vi "Do.vi"(8 "error in (no error)":errorcluster, 10 "Actor in":refnum<class "Actor.lvclass">, 11 "Linear Actuator Control Task Msg":refnum<class "Linear Actuator Control Task Msg.lvclass">) -> (0 "error out":errorcluster, 2 "Actor out":refnum<class "Actor.lvclass">)   [LabVIEW 2018, in "Linear Actuator Control Actor.lvlib" / "Linear Actuator Control Task Msg.lvclass"]
uses:
  Linear Actuator Control Task Msg.lvclass
  <vilib>/ActorFramework/Actor/Actor.lvclass
  Linear Actuator Control/Linear Actuator Control.lvclass
  C:/Program Files (x86)/National Instruments/LabVIEW 2018/vi.lib/ActorFramework/Actor/Actor.lvclass
  Linear Actuator Control Task Msg.lvclass/Linear Actuator Control Task Msg.ctl
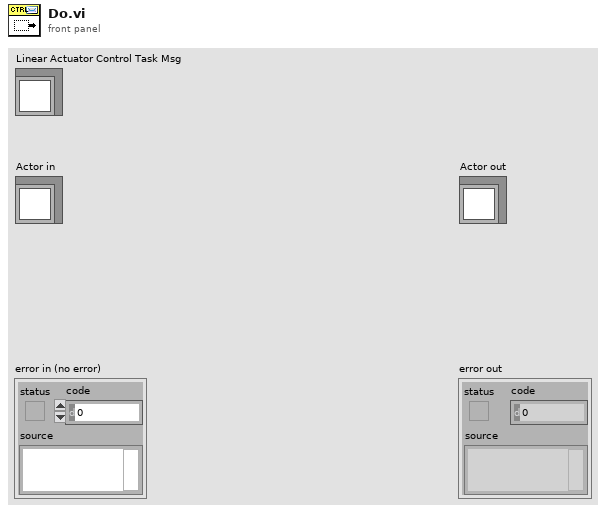
[diagram p1: front panel]
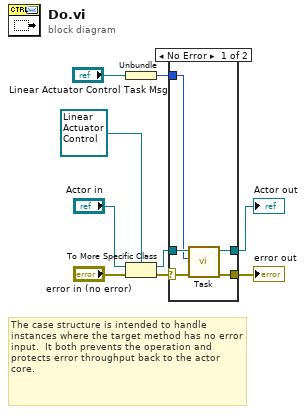
[diagram p0: block diagram]
diagram:
  # "The case structure is intended to handle instances where the target method has no error input.  It both prevents the operation and protects error throughput back to the actor core."
  n1 = Unbundle("Linear Actuator Control Task Msg") -> (w1:i32)
  n2 = To More Specific Class(target class=refnum<class "Linear Actuator Control.lvclass"> refnum ("Actor in"), reference="Actor in", error in="error in (no error)") -> (specific class reference=w8:refnum<class "Linear Actuator Control.lvclass">, error out=w4:errorcluster)
  n3 = case shown="No Error" w4 {
    selector: w4 -> [w11 w16]
    tunnel: w8 -> [w14 w15]
    tunnel: [w13 w16] -> w3
    tunnel: [w12 w15] -> w2
    tunnel: w1 -> [w10 _]
    frame No Error {
      n4 = call-dynamic "Task.vi"("error in (no error)"=w11, "Data"=w10, "Linear Actuator Control in"=w14) -> ("error out"=w13:errorcluster, "Linear Actuator Control out"=w12:refnum<class "Linear Actuator Control.lvclass">)  [unwired: 7 in]
    }
    frame Error {
    }
  }
  "error out" <- w3
  "Actor out" <- w2
